vi "Create_Run_Dir_Gain.vi"(8 "Folder name":string, 11 "Run":string) -> (3 "dup path":path)   [LabVIEW 2019]
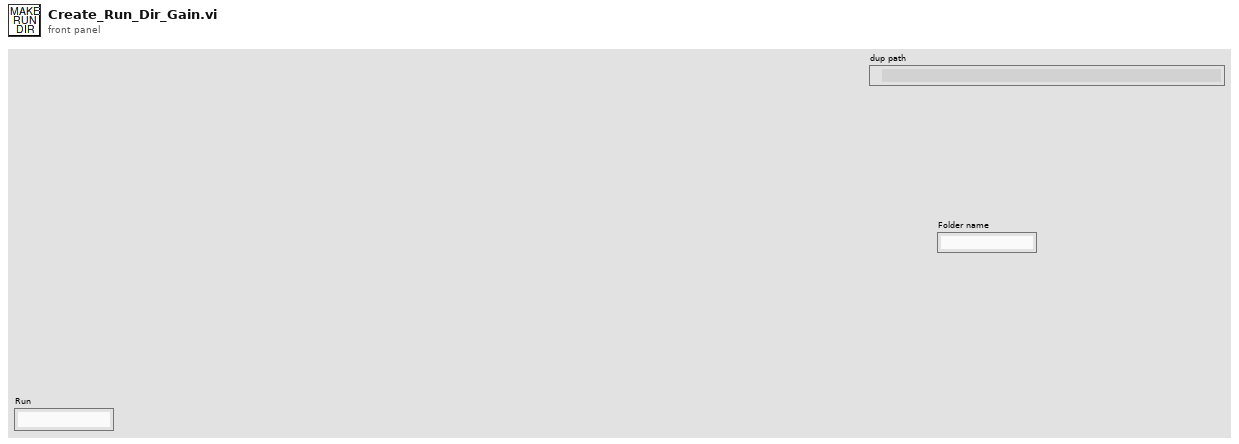
[diagram p1: front panel]
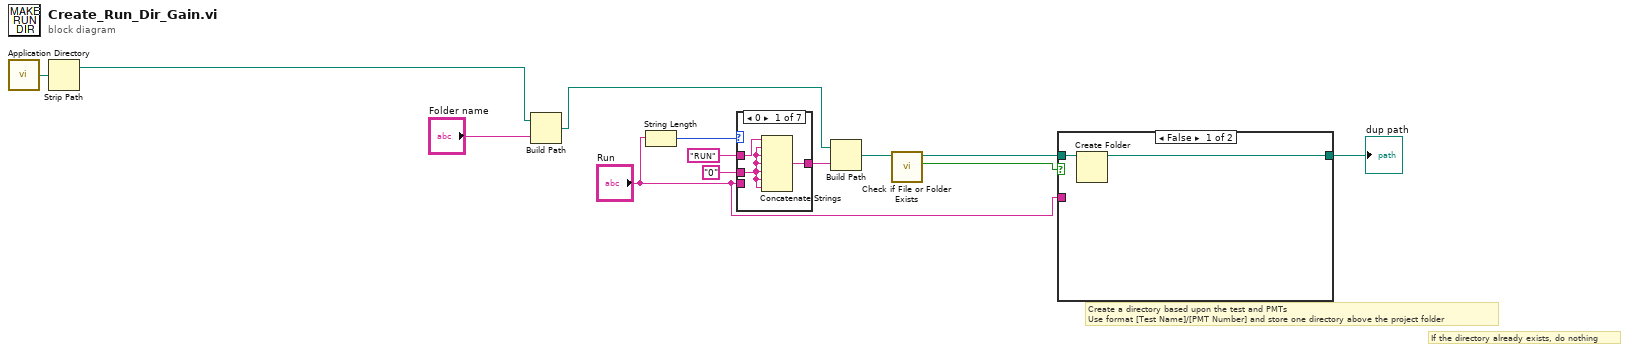
[diagram p0: block diagram]
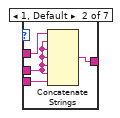
[diagram p2: hidden frame]
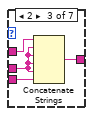
[diagram p3: hidden frame]
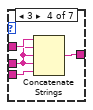
[diagram p4: hidden frame]
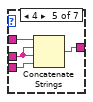
[diagram p5: hidden frame]
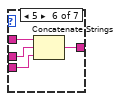
[diagram p6: hidden frame]
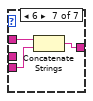
[diagram p7: hidden frame]
diagram:
  # "If the directory already exists, do nothing"
  # "Create a directory based upon the test and PMTs\nUse format [Test Name]/[PMT Number] and store one directory above the project folder"
  n1 = call <vilib>:"Application Directory.vi"() -> ("Application Directory"=w13:path)
  n2 = Strip Path(path=w13) -> (stripped path=w2:path)  [unwired: 1 out]
  n3 = Build Path(base path=w2, name or relative path="Folder name") -> (appended path=w3:path)
  n4 = String Length(string="Run") -> (length=w8:i32)
  n5 = case shown="0" w8 {
    tunnel: "RUN" ("string") -> [w16 w20 w23 w28 w31 w35 w38]
    tunnel: [w14 w19 w24 w25 w32 w36 w39] -> w6
    tunnel: "Run" -> [_ w18 w21 w26 w29 w33 w37]
    tunnel: "0" ("string") -> [w15 w17 w22 w27 w30 w34 _]
    frame 0 {
      n6 = Concatenate Strings(w16, w15, w15, w15, w15, w15, w15) -> (w14:string)
    }
    frame 1, Default {
      n7 = Concatenate Strings(w20, w17, w17, w17, w17, w17, w18) -> (w19:string)
    }
    frame 2 {
      n8 = Concatenate Strings(w23, w22, w22, w22, w22, w21) -> (w24:string)
    }
    frame 3 {
      n9 = Concatenate Strings(w28, w27, w27, w27, w26) -> (w25:string)
    }
    frame 4 {
      n10 = Concatenate Strings(w31, w30, w30, w29) -> (w32:string)
    }
    frame 5 {
      n11 = Concatenate Strings(w35, w34, w33) -> (w36:string)
    }
    frame 6 {
      n12 = Concatenate Strings(w38, w37) -> (w39:string)
    }
  }
  n13 = Build Path(base path=w3, name or relative path=w6) -> (appended path=w9:path)
  n14 = call <vilib>:"Check if File or Folder Exists.vi"("path"=w9) -> ("file or folder exists?"=w12:bool, "dup path"=w11:path)  [unwired: 8 in, 1 out]
  n15 = case shown="False" w12 {
    tunnel: w11 -> [w41 w42]
    tunnel: [w40 w42] -> w10
    tunnel: "Run" -> [_ _]
    frame False {
      n16 = Create Folder(path (use dialog)=w41) -> (created path=w40:path)  [unwired: 2 in, 2 out]
    }
    frame True {
    }
  }
  "dup path" <- w10
